vi "ORS_CursorToCropIdxRel.vi"(8 "relative index offset":i32=2, 9 "cursor index offset":i32, 11 "Cursor List":T1) -> (0 "length":i32, 1 "offset":i32)   [LabVIEW 2016]
uses:
  <vilib>/Utility/miscctls.llb/LVCursorListTypeDef.ctl
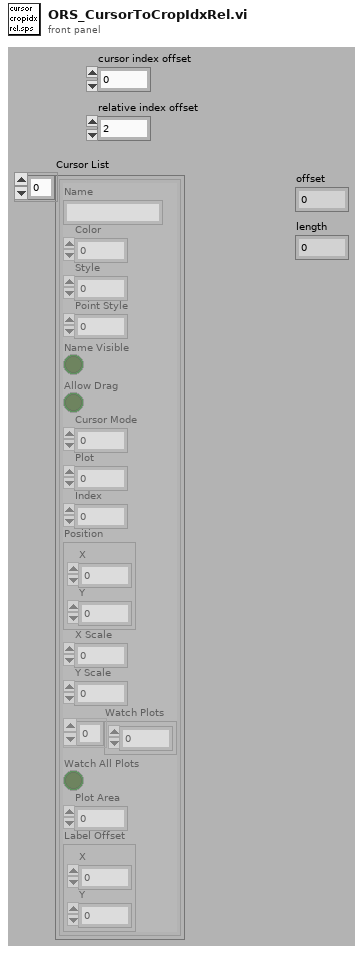
[diagram p1: front panel]
types:
  T1 = typedef "LVCursorListTypeDef.ctl" = cluster{"Name":string, "Color":u32, "Style":u8, "Point Style":u8, "Name Visible":bool, "Allow Drag":bool, "Cursor Mode":u32, "Plot":i32, "Index":i32, "Position":cluster{"X":dbl, "Y":dbl}, "X Scale":u32, "Y Scale":u32, "Watch Plots":i32[], "Watch All Plots":bool, "Plot Area":i32, "Label Offset":cluster{"X":dbl, "Y":dbl}}[]
  T2 = cluster{"Name":string, "Color":u32, "Style":u8, "Point Style":u8, "Name Visible":bool, "Allow Drag":bool, "Cursor Mode":u32, "Plot":i32, "Index":i32, "Position":cluster{"X":dbl, "Y":dbl}, "X Scale":u32, "Y Scale":u32, "Watch Plots":i32[], "Watch All Plots":bool, "Plot Area":i32, "Label Offset":cluster{"X":dbl, "Y":dbl}}
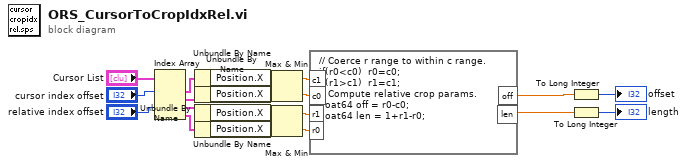
[diagram p0: block diagram]
diagram:
  n1 = Index Array(array="Cursor List", index #1="cursor index offset", index #3="relative index offset") -> (element #1=w19:T2, element #2=w18:T2, element #3=w8:T2, element #4=w7:T2)  [unwired: 2 in]
  n2 = Unbundle By Name(w19) -> ("Position.X"=w17:dbl)
  n3 = Unbundle By Name(w18) -> ("Position.X"=w16:dbl)
  n4 = Unbundle By Name(w8) -> ("Position.X"=w9:dbl)
  n5 = Unbundle By Name(w7) -> ("Position.X"=w10:dbl)
  n6 = Max & Min(x=w17, y=w16) -> (max(x,y)=w3:dbl, min(x,y)=w4:dbl)
  n7 = Max & Min(x=w9, y=w10) -> (max(x,y)=w6:dbl, min(x,y)=w5:dbl)
  n8 = formula code="// Coerce r range to within c range. \nif(r0<c0)  r0=c0;\nif(r1>c1)  r1=c1;\n// Compute relative crop params.\nfloat64 off = r0-c0;\nfloat64 len = 1+r1-r0;"("c1"=w3, "c0"=w4, "r1"=w6, "r0"=w5) -> ("off"=w2:dbl, "len"=w1:dbl)
  n9 = To Long Integer(number=w2) -> (32bit integer=→"offset":i32)
  n10 = To Long Integer(number=w1) -> (32bit integer=→"length":i32)
